vi "Tosca-Setup Schedule.vi"(0 "Tosca":refnum<class "Parameters.lvclass">) -> (4 "Tosca out":refnum<class "Parameters.lvclass">, 8 "Canceled?":bool)   [LabVIEW 2020]
uses:
  epl-vi-lib/Utility VIs/Controls/KTable/KTable.xctl
  epl-vi-lib/Utility VIs/Buttons/KCheckmarkBoolean 2.ctl
  epl-vi-lib/Utility VIs/Controls/KListboxEx/KListboxEx.xctl
  Classes/Parameters/Parameters.lvclass
  epl-vi-lib/Utility VIs/Controls/KTable/Events.ctl
  epl-vi-lib/Utility VIs/Controls/KTable/Event Data.ctl
  epl-vi-lib/Utility VIs/Controls/KTable/Event Type.ctl
  <vilib>/Utility/miscctls.llb/LVPoint32TypeDef.ctl
  epl-vi-lib/Utility VIs/Controls/KListboxEx/Event Action.ctl
  Typedefs/Tosca-Schedule Mode.ctl
  Classes/Parameters/Parameters.lvclass/Parameters.ctl
  Typedefs/Tosca-Adaptive Track.ctl
  Typedefs/Tosca-Simple Variable.ctl
  Adaptation VIs/Tosca-Adapt Threshold Metric.ctl
  Typedefs/Tosca-Parameter Family.ctl
  Typedefs/Tosca-Parameter Table Element.ctl
  Typedefs/Tosca-Parameter Dimension.ctl
  Typedefs/Tosca-Sequence Order.ctl
  Classes/Parameters/Read Schedule Mode.vi
  Classes/Parameters/Read Schedule.vi
  Classes/Parameters/Write Tracks.vi
  Classes/Parameters/Read Tracks.vi
  Classes/Parameters/Write Schedule Mode.vi
  Classes/Parameters/Write Schedule.vi
  Classes/Parameters/Read Families.vi
  Classes/Parameters/Write Families.vi
  Classes/Parameters/Read Adapt.vi
  Classes/Parameters/Write Adapt.vi
panel:
  in  "icon":u16(ring)
  in  "Mode":u16(ring) caption="Configure as" items=["Sequence", "CS+/CS-", "Adaptive track"]
  in  "OK":bool
  in  "Cancel":bool
  in  "Tab Control":enum32{"Schedule", "Adapt"}(tab)
  in  "browse":bool
  in  "Script":string
  in  "Update":bool
  in  "Balance":T1
  in  "order":u16(ring) items=["Sequential", "Alternate", "Randomized", "Random group", "Arbitrary"]
  in  "Family":u16(xcontrol)
  in  "Params":u16(xcontrol) caption="Parameters to vary for \"Item1\""
  out "Grid":i32[][](graph)
  in  "Blocks":i32 caption="Do this many blocks"
  in  "Test param":u16(xcontrol) caption="Test parameters"
  in  "switch type":enum16{"Trials", "Reversals"}(ring)
  in  "Switch after":i32
  in  "all catch":T1 caption="Do all catch"
  in  "Tracks":i32(xcontrol)
  in  "Pcatch":dbl caption="Probability of catch trial"
  in  "Adapt":T2={"mode"=enum."Add", "Step"="", "Start"=0.0, "Min"=0.0, "Max"=0.0, "Nup"=0, "Ndown"=0, "Nrev"=0, "compute"=enum."mean", "Ncompute"=0, "Step2"="", "change after"=1}
  in  "Catch parameters":u16(xcontrol) caption="Use 'A' for current value"
  in  "Adapt param":u16(xcontrol) caption="Stimulus"
  # "reversals"
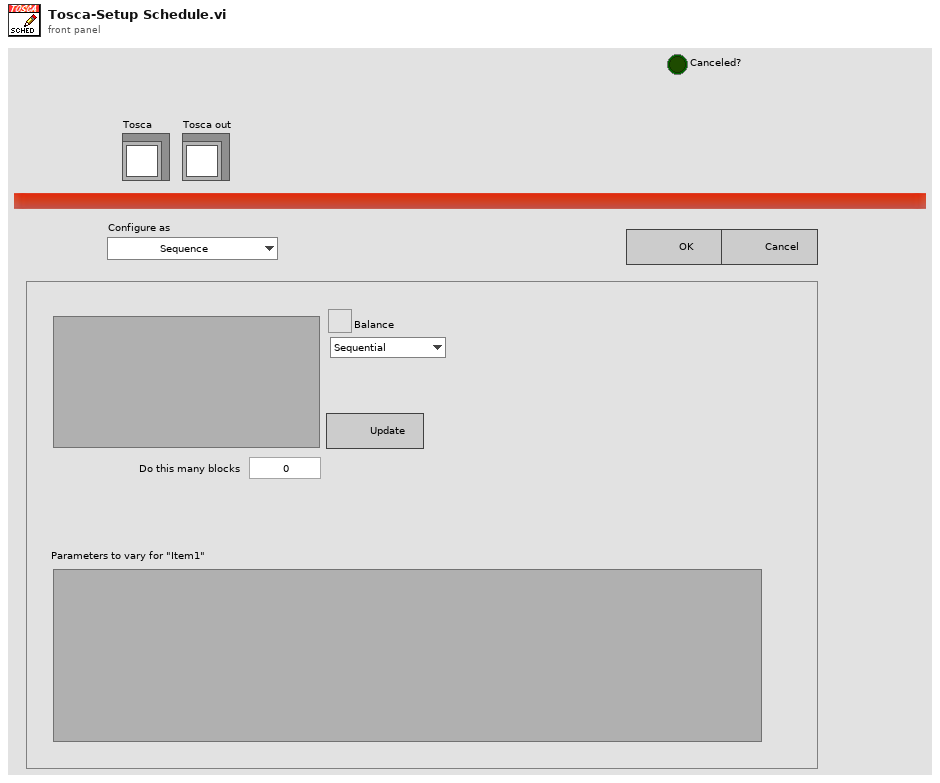
[diagram p1: front panel]
types:
  T1 = typedef "KCheckmarkBoolean 2.ctl" = bool
  T2 = cluster{"mode":enum16{"Add", "Multiply"}, "Step":string, "Start":dbl, "Min":dbl, "Max":dbl, "Nup":i32, "Ndown":i32, "Nrev":i32, "compute":enum16{"mean", "median"}, "Ncompute":i32, "Step2":string, "change after":i32}
  T3 = typedef "KTable.xctl/Events.ctl" = cluster{"Items Changed":refnum<user-event>}
  T4 = cluster{"Items Changed":refnum<user-event>, "List Changed":refnum<user-event>}
  T5 = typedef "LVPoint32TypeDef.ctl" = cluster{"Horizontal":i32, "Vertical":i32}
  T6 = cluster{"Coords":T5, "mouse":bool, "labels":string[][]}
  T7 = typedef "KListboxEx.xctl/Events.ctl" = cluster{"Items Changed":refnum<user-event>, "List Changed":refnum<user-event>}
  T8 = typedef "Tosca-Schedule Mode.ctl" = enum16{"Seq", "CS+/CS-", "Adapt"}
  T9 = typedef "Tosca-Adaptive Track.ctl" = cluster{"state":string, "chan":string, "param":string, "Start":dbl, "Step":string, "Mode":enum16{"Add", "Multiply"}, "Pcatch":dbl, "Ndown":i32, "Nup":i32, "Nreverse":i32, "Min":dbl, "Max":dbl, "Catch":T10[], "do all catch":bool, "name":string, "Vars":T10[], "compute":T11, "of last":i32, "Step2":string, "after":i32}
  T10 = typedef "Tosca-Simple Variable.ctl" = cluster{"state":string, "chan":string, "param":string, "expr":string}
  T11 = typedef "Tosca-Adapt Threshold Metric.ctl" = enum16{"mean", "median"}
  T12 = typedef "Tosca-Parameter Family.ctl" = cluster{"Name":string, "Number":i32, "Vars":T13[], "Mask":bool[][], "one each":bool}
  T13 = typedef "Tosca-Parameter Table Element.ctl" = cluster{"state":string, "chan":string, "param":string, "expr":string, "dim":T14, "value":dbl[]}
  T14 = typedef "Tosca-Parameter Dimension.ctl" = enum16{"Ind", "X", "Y"}
  T15 = typedef "Tosca-Sequence Order.ctl" = enum16{"Sequential", "Alternate", "Randomize", "Random group", "Arbitrary"}
  T16 = typedef "Tosca-Schedule.ctl" = cluster{"Blocks":i32, "order":T15, "balance":bool, "Families":T12[], "Script":path}
  T17 = typedef "KTable.xctl/Event Type.ctl" = enum16{"None", "Selection", "Edit", "Insert", "Delete", "Up", "Down", "Duplicate"}
  T18 = typedef "KListboxEx.xctl/Event Action.ctl" = enum16{"None", "Add", "Delete", "Move", "Edit", "Select"}
  T19 = typedef "Tosca-Adapt.ctl" = cluster{"Switch after":i32, "Switch type":enum16{"Trials", "Reversals"}, "Tracks":T9[]}
  T20 = cluster{"state":string, "chan":string, "param":string}[]
  T21 = cluster{"state":string, "chan":string, "param":string}
  T22 = cluster{"state":string, "chan":string, "param":string, "expr":string}[]
  T23 = cluster{"Name":string, "Number":i32, "one each":bool}
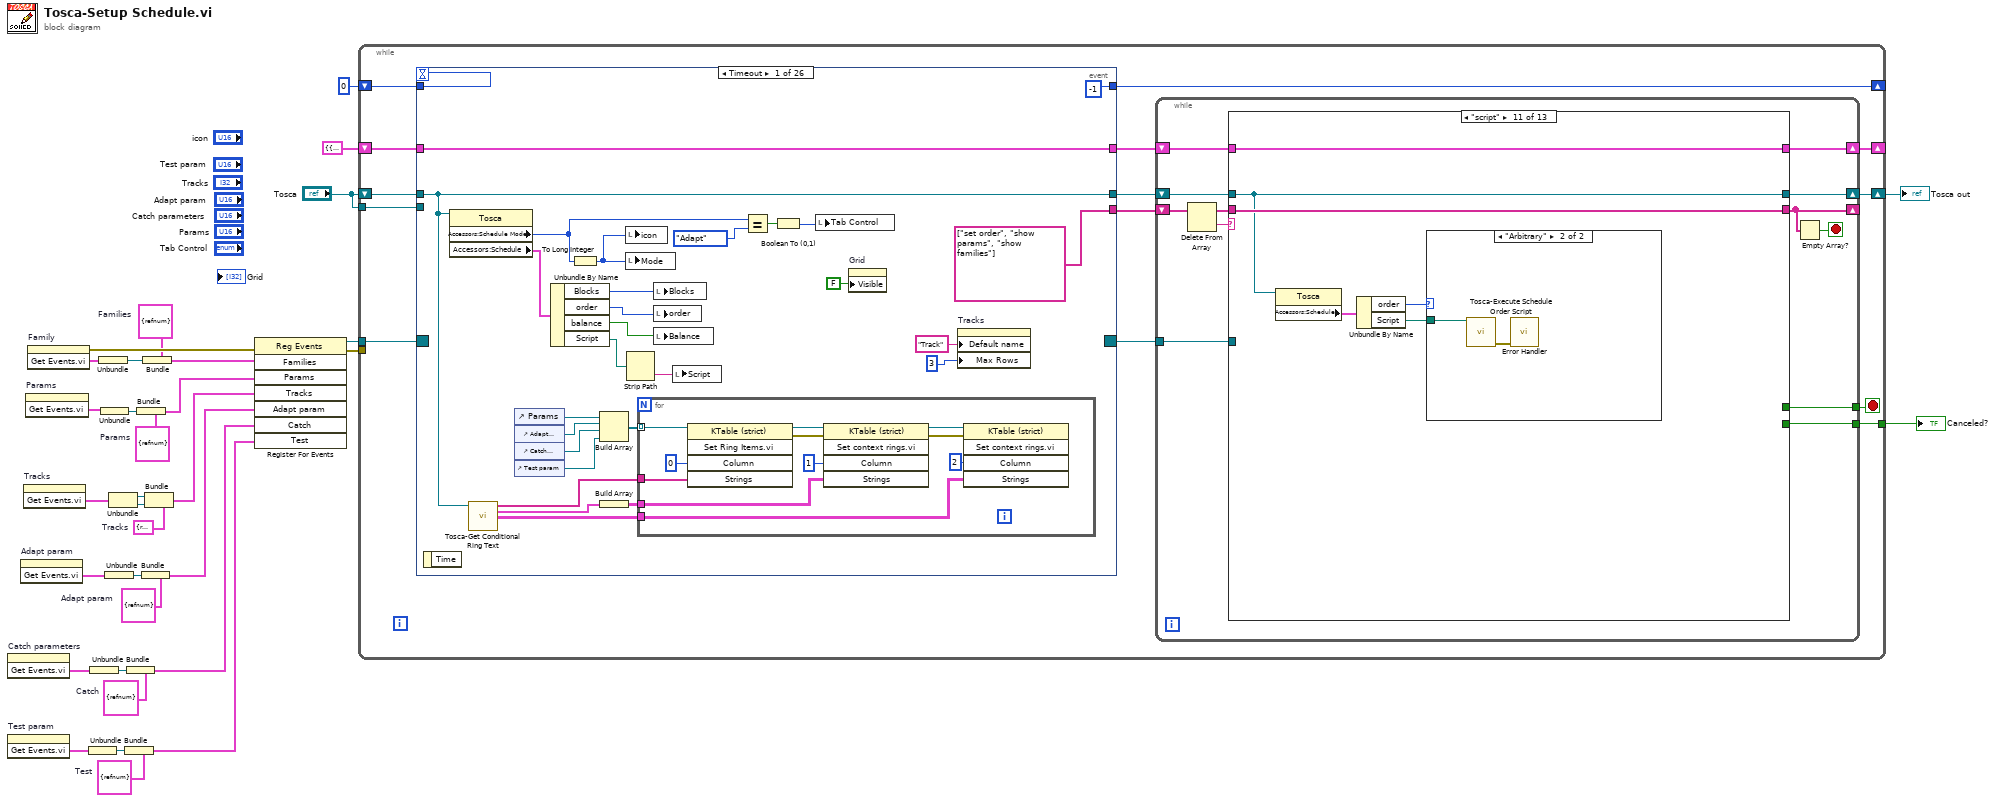
[diagram p0: block diagram]
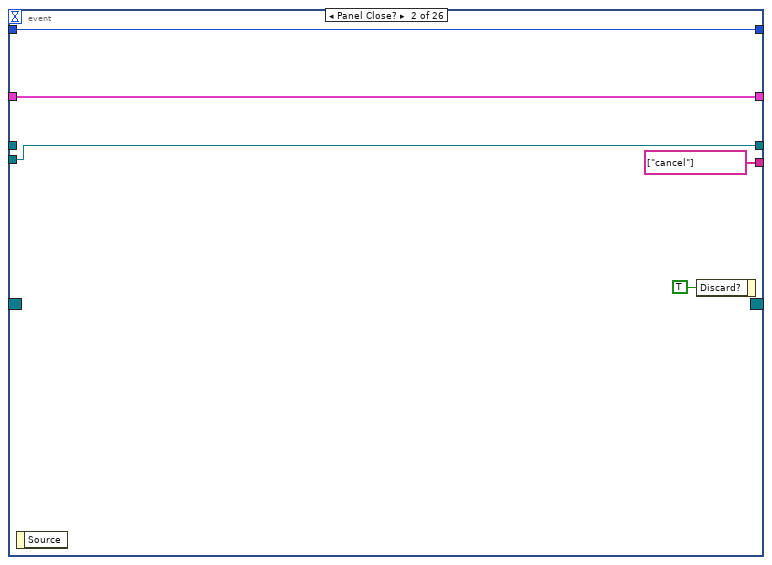
[diagram p2: hidden frame]
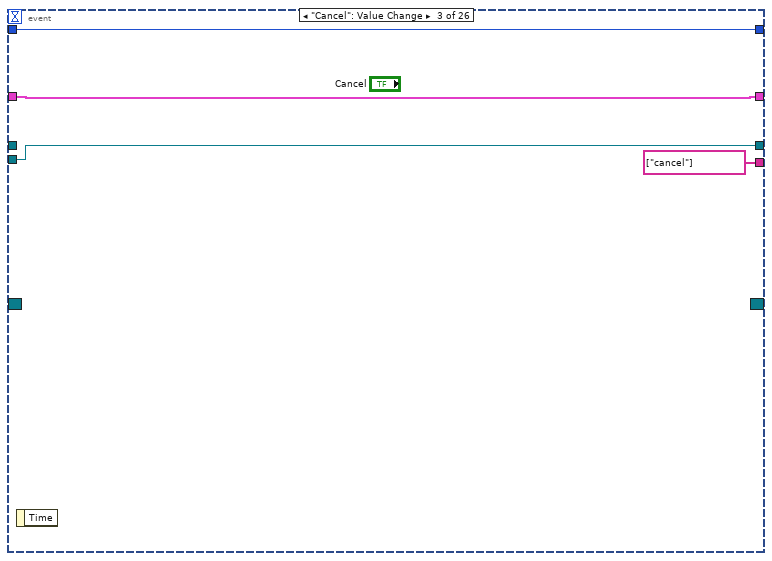
[diagram p3: hidden frame]
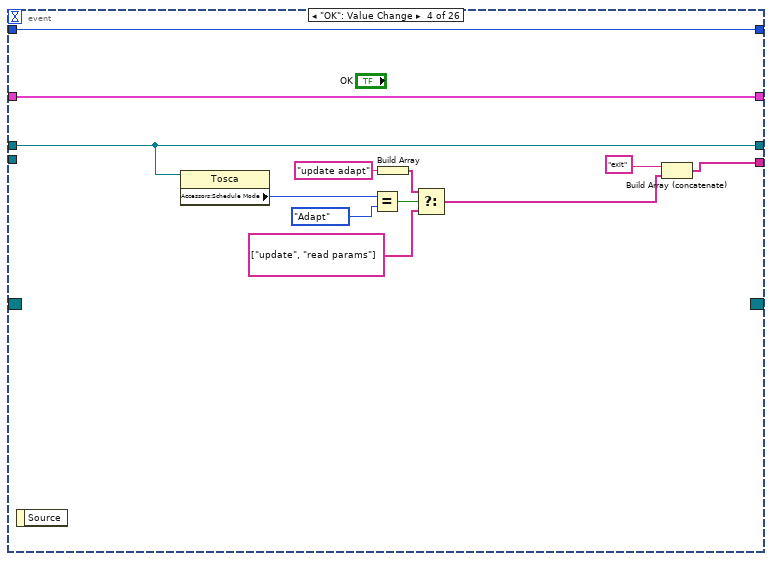
[diagram p4: hidden frame]
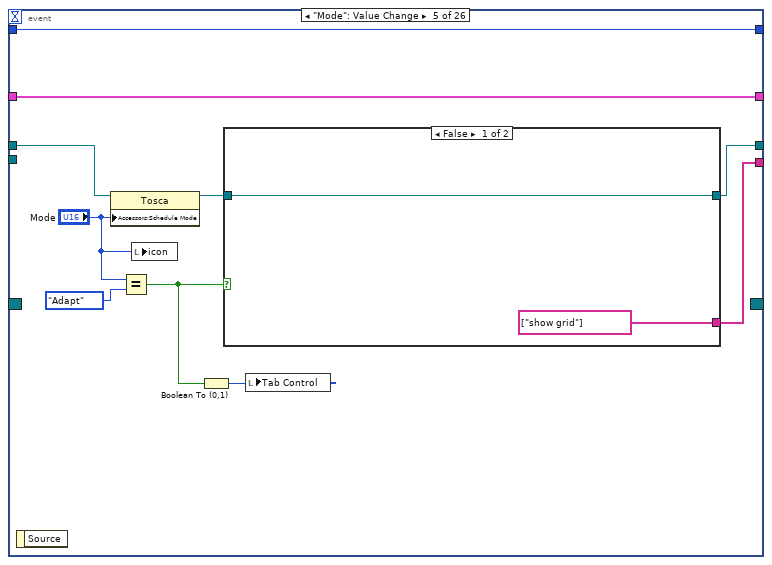
[diagram p5: hidden frame]
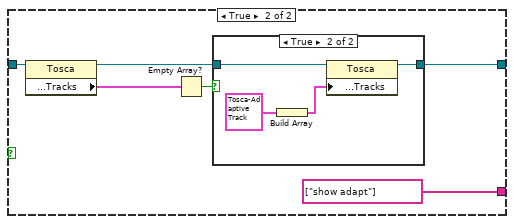
[diagram p6: hidden frame]
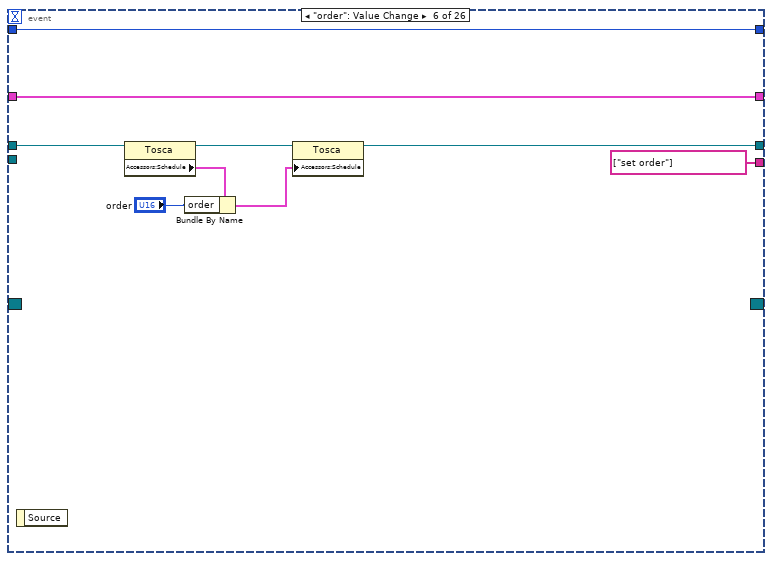
[diagram p8: hidden frame]
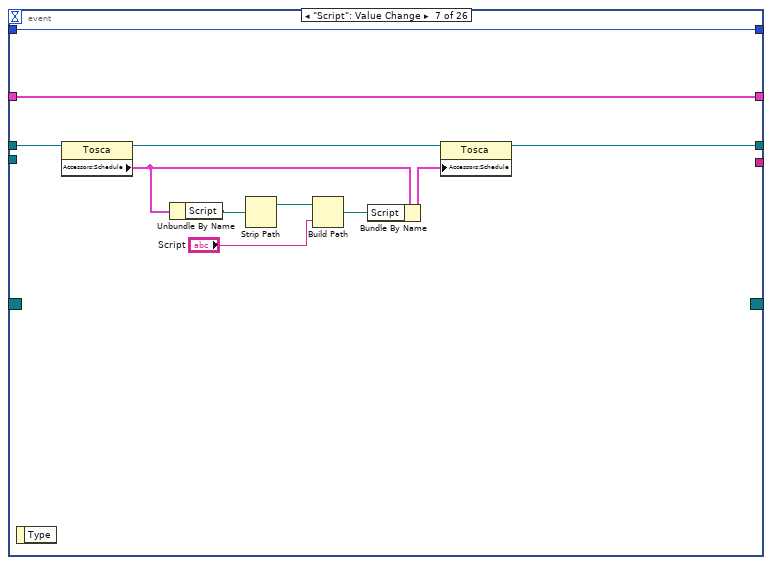
[diagram p9: hidden frame]
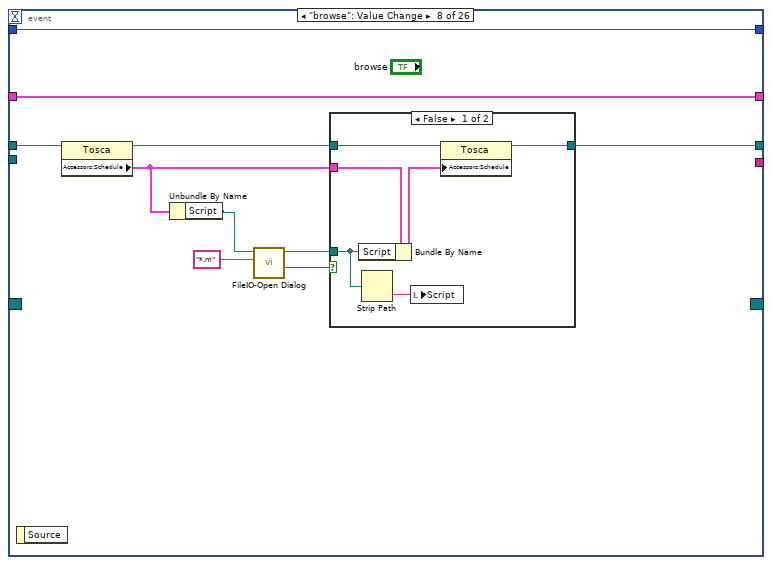
[diagram p10: hidden frame]
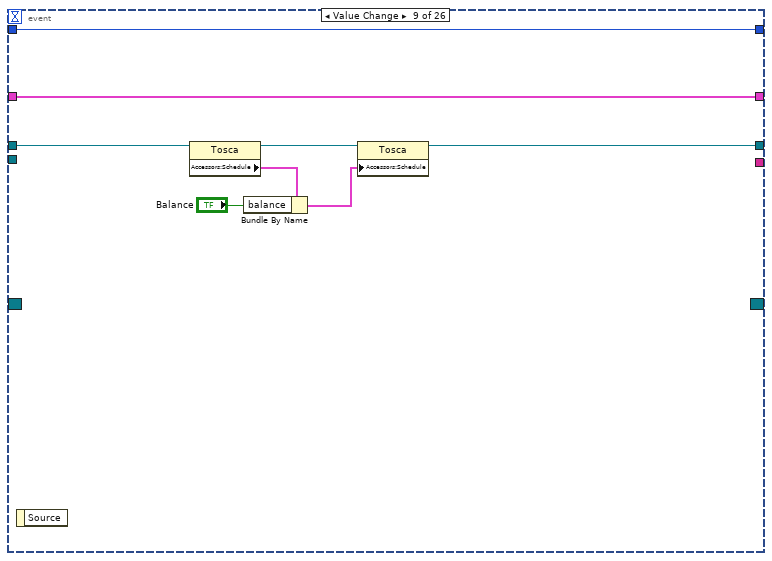
[diagram p12: hidden frame]
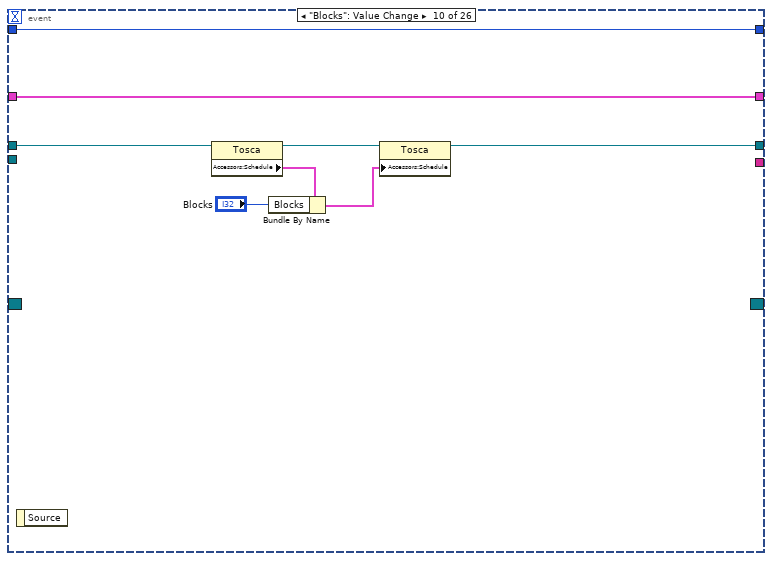
[diagram p13: hidden frame]
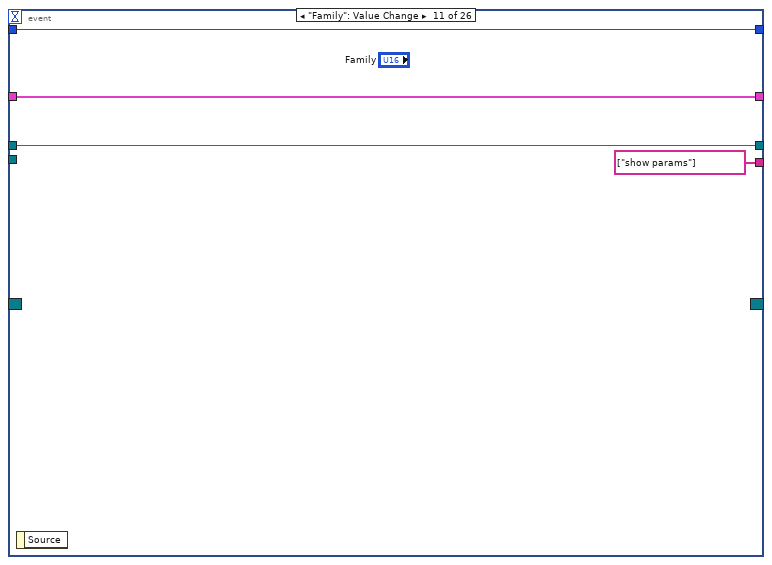
[diagram p14: hidden frame]
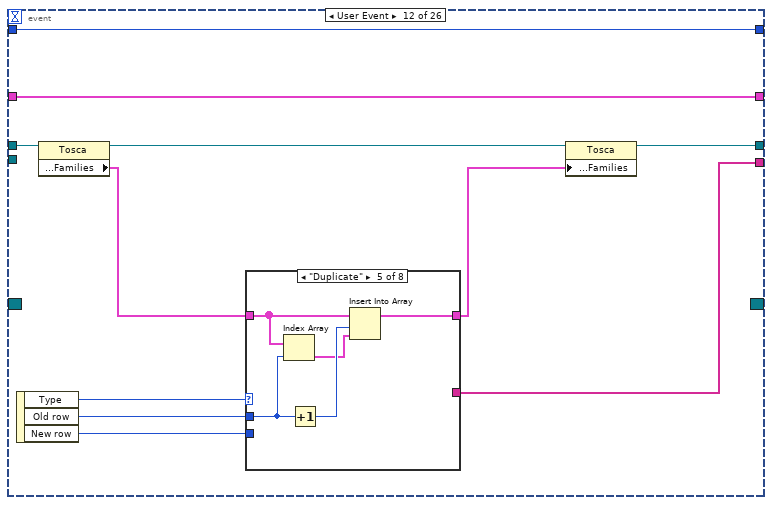
[diagram p15: hidden frame]
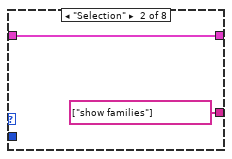
[diagram p17: hidden frame]
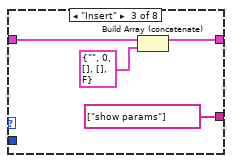
[diagram p18: hidden frame]
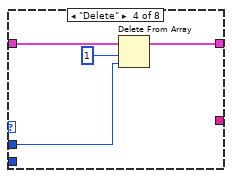
[diagram p19: hidden frame]
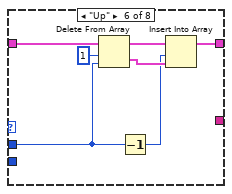
[diagram p20: hidden frame]
diagram:
  w7 = T3 {"Items Changed"=refnum}  # Test
  w10 = T3 {"Items Changed"=refnum}  # Catch
  w14 = T3 {"Items Changed"=refnum}  # Adapt param
  w17 = T4 {"Items Changed"=refnum, "List Changed"=refnum}  # Tracks
  w24 = T3 {"Items Changed"=refnum}  # Params
  w30 = T3 {"Items Changed"=refnum}  # Families
  n1 = invoke on="Catch parameters" class="KTable (strict)" method="Get Events.vi"() -> ("Get Events.vi"=w11:T3)  [unwired: 3 in, 2 out]
  n2 = invoke on="Test param" class="KTable (strict)" method="Get Events.vi"() -> ("Get Events.vi"=w6:T3)  [unwired: 3 in, 2 out]
  n3 = invoke on="Adapt param" class="KTable (strict)" method="Get Events.vi"() -> ("Get Events.vi"=w15:T3)  [unwired: 3 in, 2 out]
  n4 = invoke on="Tracks" class="KListboxEx (strict)" method="Get Events.vi"() -> ("Get Events.vi"=w20:T7)  [unwired: 3 in, 2 out]
  n5 = invoke on="Params" class="KTable (strict)" method="Get Events.vi"() -> ("Get Events.vi"=w25:T3)  [unwired: 3 in, 2 out]
  n6 = invoke on="Family" class="KTable (strict)" method="Get Events.vi"() -> (error out=w31:errorcluster, "Get Events.vi"=w29:T3)  [unwired: 3 in, 1 out]
  n7 = Unbundle(w6) -> ("Items Changed"=w8:refnum<user-event>)
  n8 = Unbundle(w11) -> ("Items Changed"=w12:refnum<user-event>)
  n9 = Unbundle(w29) -> ("Items Changed"=w28:refnum<user-event>)
  n10 = Unbundle(w25) -> ("Items Changed"=w26:refnum<user-event>)
  n11 = Unbundle(w15) -> ("Items Changed"=w16:refnum<user-event>)
  n12 = Unbundle(w20) -> ("Items Changed"=w21:refnum<user-event>, "List Changed"=w19:refnum<user-event>)
  n13 = Bundle(cluster=w7, "Items Changed"=w8) -> (w5:T3)
  n14 = Bundle(cluster=w10, "Items Changed"=w12) -> (w9:T3)
  n15 = Bundle(cluster=w24, "Items Changed"=w26) -> (w23:T3)
  n16 = Bundle(cluster=w14, "Items Changed"=w16) -> (w13:T3)
  n17 = Bundle(cluster=w30, "Items Changed"=w28) -> (w27:T3)
  n18 = Bundle(cluster=w17, "Items Changed"=w21, "List Changed"=w19) -> (w18:T4)
  n19 = register-events(error in=w31, w27, w23, w18, w13, w9, w5) -> (reference out=w1:refnum<event-registration>, error out=w2:errorcluster)  [unwired: 1 in]
  n20 = while {
    shift-right: [w47] -> _
    shift-left: 0 -> [w46]
    tunnel: [w39] -> w32
    shift-right: [w41] -> w3
    shift-left: "Tosca" -> [w45]
    tunnel: "Tosca" -> [w44]
    shift-right: [w36] -> _
    shift-left: T6 {"Coords"={"Horizontal"=0, "Vertical"=0}, "mouse"=FALSE, "labels"=[]} -> [w38]
    tunnel: w2 -> [_]
    tunnel: w1 -> [w35]
    stop <- w40 stop-if-true
    n21 = event shown="[0] Timeout" {
      selector: w35 -> [_ _ _ _ _ _ _ _ _ _ _ _ _ _ _ _ _ _ _ _ _ _ _ _ _ _]
      dyn-events: [_ _ _ _ _ _ _ _ _ _ _ _ _ _ _ _ _ _ _ _ _ _ _ _ _ _] -> w34
      timeout: w46 -> [_ _ _ _ _ _ _ _ _ _ _ _ _ _ _ _ _ _ _ _ _ _ _ _ _ _]
      tunnel: [-1 w90 w94 w106 w116 w138 w149 w159 w174 w182 w186 w197 w241 w284 w299 w314 w336 w373 w382 w390 w414 w425 w442 w455 w468 w479] -> w47
      tunnel: w46 -> [_ w90 w94 w106 w116 w138 w149 w159 w174 w182 w186 w197 w241 w284 w299 w314 w336 w373 w382 w390 w414 w425 w442 w455 w468 w479]
      tunnel: w45 -> [w50 _ _ w96 w110 w135 w147 w157 w169 w176 w185 w190 w234 w283 w296 w304 w329 w367 w379 w384 w395 w419 w430 w447 w460 w473]
      tunnel: [w50 w86 w93 w96 w107 w131 w140 w154 w168 w175 w185 w189 w233 w283 w296 w303 w325 w366 w377 w383 w394 w418 w428 w446 w459 w472] -> w43
      tunnel: w44 -> [_ w86 w93 _ _ _ _ _ _ _ _ _ _ _ _ _ _ _ _ _ _ _ _ _ _ _]
      tunnel: [string[] ["set order", "show params", "show families"] string[] ["cancel"] string[] ["cancel"] w102 w112 string[] ["set order"] _ _ _ _ string[] ["show params"] w193 w237 string[] ["script", "update", "read params"] _ _ w330 w371 _ _ _ _ _ _ _ _] -> w42
      tunnel: w38 -> [w66 w89 w91 w105 w115 w136 w148 w158 w173 w181 w184 w192 w235 w281 w291 w305 w335 w372 w381 w389 w413 w424 w441 w454 w467 w478]
      tunnel: [w66 w89 w91 w105 w115 w136 w148 w158 w173 w181 w184 w192 w235 w281 w289 w305 w335 w372 w381 w389 w413 w424 w441 w454 w467 w478] -> w37
      event Timeout {
        n22 = event-data() -> ()  [unwired: 1 in, 1 out]
        n23 = property class="Tosca"(reference=w50) -> ("Accessors:Schedule Mode"=w51:T8, "Accessors:Schedule"=w52:T16)  [unwired: 1 in, 2 out]
        n24 = call "Tosca-Get Conditional Ring Text.vi"("Tosca"=w50) -> ("States"=w53:string[], "StimChans"=w73:cluster{string[]}[], "Params"=w71:cluster{"Parameter Names":string[]}[][])  [unwired: 12 in]
        n25 = control-ref of="Params"() -> (w60:refnum<vi>)
        n26 = control-ref of="Adapt param"() -> (w59:refnum<vi>)
        n27 = control-ref of="Catch parameters"() -> (w58:refnum<vi>)
        n28 = control-ref of="Test param"() -> (w54:refnum<vi>)
        n29 = Unbundle By Name(w52) -> ("Blocks"=w70:i32, "order"=w69:T15, "balance"=w68:bool, "Script"=w49:path)
        n30 = To Long Integer(number=w51) -> (32bit integer=w65:i32)
        n31 = Build Array(w60, w59, w58, w54) -> (w57:refnum<vi>[])
        n32 = Build Array(w73) -> (w72:cluster{string[]}[][])
        n33 = local write "icon"(w65) -> ()
        n34 = local write "Mode"(w65) -> ()
        n35 = Strip Path(path=w49) -> (name=w48:string)  [unwired: 1 out]
        n36 = for {
          tunnel: w72 -> [w80]
          tunnel: w71 -> [w79]
          tunnel: w53 -> [w78]
          tunnel: w57 -> [w75] mode=indexing
          n37 = invoke on="Invoke Node" class="KTable (strict)" method="Set Ring Items.vi"(reference=w75, "Column"=0, "Strings"=w78) -> (reference out=w77:refnum<vi>, error out=w83:errorcluster)  [unwired: 2 in, 3 out]
          n38 = invoke on="Invoke Node" class="KTable (strict)" method="Set context rings.vi"(reference=w77, error in=w83, "Column"=1, "Strings"=w80) -> (reference out=w76:refnum<vi>, error out=w82:errorcluster)  [unwired: 1 in, 3 out]
          n39 = invoke on="Invoke Node" class="KTable (strict)" method="Set context rings.vi"(reference=w76, error in=w82, "Column"=2, "Strings"=w79) -> ()  [unwired: 1 in, 5 out]
        }
        n40 = local write "Blocks"(w70) -> ()
        n41 = local write "order"(w69) -> ()
        n42 = local write "Balance"(w68) -> ()
        n43 = local write "Script"(w48) -> ()
        n44 = Equal?(x=w51, y=Tosca-Schedule_Mode."Adapt") -> (x = y?=w63:bool)
        n45 = Boolean To (0,1)(Boolean=w63) -> (0, 1=w62:i16)
        n46 = local write "Tab Control"(w62) -> ()
        n47 = property on="Grid" class="IntGraph (strict)"("Visible"=FALSE) -> ()  [unwired: 2 in, 2 out]
        n48 = property on="Tracks" class="KListboxEx (strict)"("Default name"="Track", "Max Rows"=3) -> ()  [unwired: 2 in, 2 out]
      }
      event Panel Close? {
        n49 = event-data() -> ()  [unwired: 1 in, 1 out]
        n50 = event-data("Discard?"=TRUE) -> ()  [unwired: 1 in, 1 out]
      }
      event "Cancel": Value Change {
        n51 = event-data() -> ()  [unwired: 1 in, 1 out]
      }
      event "OK": Value Change {
        n52 = event-data() -> ()  [unwired: 1 in, 1 out]
        n53 = property class="Tosca"(reference=w96) -> ("Accessors:Schedule Mode"=w95:T8)  [unwired: 1 in, 2 out]
        n54 = Equal?(x=w95, y=Tosca-Schedule_Mode."Adapt") -> (x = y?=w100:bool)
        n55 = Build Array("update adapt" ("t")) -> (w98:string[])
        n56 = Select(t=w98, s=w100, f=string[] ["update", "read params"]) -> (s? t:f=w103:string[])
        n57 = Build Array (concatenate)("exit", w103) -> (w102:string[])
      }
      event "Mode": Value Change {
        n58 = event-data() -> ()  [unwired: 1 in, 1 out]
        n59 = property class="Tosca"(reference=w110, "Accessors:Schedule Mode"="Mode") -> (reference out=w108:refnum<class "Parameters.lvclass">)  [unwired: 1 in, 1 out]
        n60 = Equal?(x="Mode", y=Tosca-Schedule_Mode."Adapt") -> (x = y?=w113:bool)
        n61 = local write "icon"("Mode") -> ()
        n62 = Boolean To (0,1)(Boolean=w113) -> (0, 1=w114:i16)
        n63 = case shown="False" w113 {
          tunnel: [string[] ["show grid"] string[] ["show adapt"]] -> w112
          tunnel: w108 -> [w117 w122]
          tunnel: [w117 w119] -> w107
          frame False {
          }
          frame True {
            n64 = property class="Tosca"(reference=w122) -> (reference out=w120:refnum<class "Parameters.lvclass">, "Accessors:Adapt.Tracks"=w121:T9[])  [unwired: 1 in, 1 out]
            n65 = Empty Array?(array=w121) -> (empty?=w123:bool)
            n66 = case shown="True" w123 {
              tunnel: w120 -> [w125 w128]
              tunnel: [w125 w127] -> w119
              frame False {
              }
              frame True {
                n67 = Build Array(T9 {"state"="", "chan"="", "param"="", "Start"=90.0, "Step"="-5", "Mode"=enum."Add", "Pcatch"=100.0, "Ndown"=2, "Nup"=1, "Nreverse"=6, "Min"=0.0, "Max"=100.0, "Catch"=[], "do all catch"=FALSE, "name"="Track1", "Vars"=[], "compute"=enum."mean", "of last"=0, "Step2"="", "after"=0} ("Track")) -> (w126:T9[])
                n68 = property class="Tosca"(reference=w128, "Accessors:Adapt.Tracks"=w126) -> (reference out=w127:refnum<class "Parameters.lvclass">)  [unwired: 1 in, 1 out]
              }
            }
          }
        }
        n69 = local write "Tab Control"(w114) -> ()
      }
      event "order": Value Change {
        n70 = event-data() -> ()  [unwired: 1 in, 1 out]
        n71 = property class="Tosca"(reference=w135) -> (reference out=w133:refnum<class "Parameters.lvclass">, "Accessors:Schedule"=w134:T16)  [unwired: 1 in, 1 out]
        n72 = Bundle By Name(cluster=w134, "order"="order") -> (w132:T16)
        n73 = property class="Tosca"(reference=w133, "Accessors:Schedule"=w132) -> (reference out=w131:refnum<class "Parameters.lvclass">)  [unwired: 1 in, 1 out]
      }
      event "Script": Value Change {
        n74 = event-data() -> ()  [unwired: 1 in, 1 out]
        n75 = property class="Tosca"(reference=w147) -> (reference out=w141:refnum<class "Parameters.lvclass">, "Accessors:Schedule"=w143:T16)  [unwired: 1 in, 1 out]
        n76 = Unbundle By Name(w143) -> ("Script"=w146:path)
        n77 = Strip Path(path=w146) -> (stripped path=w145:path)  [unwired: 1 out]
        n78 = Build Path(base path=w145, name or relative path="Script") -> (appended path=w142:path)
        n79 = Bundle By Name(cluster=w143, "Script"=w142) -> (w139:T16)
        n80 = property class="Tosca"(reference=w141, "Accessors:Schedule"=w139) -> (reference out=w140:refnum<class "Parameters.lvclass">)  [unwired: 1 in, 1 out]
      }
      event "browse": Value Change {
        n81 = event-data() -> ()  [unwired: 1 in, 1 out]
        n82 = property class="Tosca"(reference=w157) -> (reference out=w155:refnum<class "Parameters.lvclass">, "Accessors:Schedule"=w156:T16)  [unwired: 1 in, 1 out]
        n83 = Unbundle By Name(w156) -> ("Script"=w153:path)
        n84 = call "FileIO-Open Dialog.vi"("pattern (all files)"="*.m", "Start path"=w153) -> ("cancelled"=w151:bool, "selected path"=w150:path)  [unwired: 7 in, 1 out]
        n85 = case shown="False" w151 {
          tunnel: w156 -> [w165 _]
          tunnel: w155 -> [w164 w166]
          tunnel: [w163 w166] -> w154
          tunnel: w150 -> [w161 _]
          frame False {
            n86 = Bundle By Name(cluster=w165, "Script"=w161) -> (w162:T16)
            n87 = Strip Path(path=w161) -> (name=w160:string)  [unwired: 1 out]
            n88 = local write "Script"(w160) -> ()
            n89 = property class="Tosca"(reference=w164, "Accessors:Schedule"=w162) -> (reference out=w163:refnum<class "Parameters.lvclass">)  [unwired: 1 in, 1 out]
          }
          frame True {
          }
        }
      }
      event Value Change {
        n90 = event-data() -> ()  [unwired: 1 in, 1 out]
        n91 = property class="Tosca"(reference=w169) -> (reference out=w171:refnum<class "Parameters.lvclass">, "Accessors:Schedule"=w172:T16)  [unwired: 1 in, 1 out]
        n92 = Bundle By Name(cluster=w172, "balance"="Balance") -> (w170:T16)
        n93 = property class="Tosca"(reference=w171, "Accessors:Schedule"=w170) -> (reference out=w168:refnum<class "Parameters.lvclass">)  [unwired: 1 in, 1 out]
      }
      event "Blocks": Value Change {
        n94 = event-data() -> ()  [unwired: 1 in, 1 out]
        n95 = property class="Tosca"(reference=w176) -> (reference out=w179:refnum<class "Parameters.lvclass">, "Accessors:Schedule"=w180:T16)  [unwired: 1 in, 1 out]
        n96 = Bundle By Name(cluster=w180, "Blocks"="Blocks") -> (w178:T16)
        n97 = property class="Tosca"(reference=w179, "Accessors:Schedule"=w178) -> (reference out=w175:refnum<class "Parameters.lvclass">)  [unwired: 1 in, 1 out]
      }
      event "Family": Value Change {
        n98 = event-data() -> ()  [unwired: 1 in, 1 out]
      }
      event User Event {
        n99 = event-data() -> ("Type"=w196:T17, "Old row"=w195:i32, "New row"=w194:i32)  [unwired: 1 in]
        n100 = property class="Tosca"(reference=w190) -> (reference out=w191:refnum<class "Parameters.lvclass">, "Accessors:Schedule.Families"=w188:T12[])  [unwired: 1 in, 1 out]
        n101 = case shown="\"Duplicate\"" w196 {
          tunnel: w195 -> [_ _ _ w207 w213 w218 w225 _]
          tunnel: [w198 w200 w204 w205 w211 w214 w221 w229] -> w187
          tunnel: w194 -> [_ _ _ _ _ _ _ _]
          tunnel: w188 -> [w198 w200 w203 w206 w212 w216 w223 w229]
          tunnel: [_ string[] ["show families"] string[] ["show params"] _ _ _ _ string[] ["show params", "read families"]] -> w193
          frame "None", Default {
          }
          frame "Selection" {
          }
          frame "Insert" {
            n102 = Build Array (concatenate)(w203, T12 {"Name"="", "Number"=0, "Vars"=[], "Mask"=[], "one each"=FALSE} ("Family")) -> (w204:T12[])
          }
          frame "Delete" {
            n103 = Delete From Array(array=w206, length=1, index=w207) -> (array with subset deleted=w205:T12[])  [unwired: 1 out]
          }
          frame "Duplicate" {
            n104 = Index Array(array=w212, index=w213) -> (element=w209:T12)
            n105 = Increment(x=w213) -> (x+1=w210:i32)
            n106 = Insert Into Array(array=w212, index=w210, new element=w209) -> (w211:T12[])
          }
          frame "Up" {
            n107 = Delete From Array(array=w216, length=1, index=w218) -> (deleted portion=w219:T12[], array with subset deleted=w215:T12[])
            n108 = Decrement(x=w218) -> (x-1=w217:i32)
            n109 = Insert Into Array(array=w215, index=w217, new element=w219) -> (w214:T12[])
          }
          frame "Down" {
            n110 = Delete From Array(array=w223, length=1, index=w225) -> (deleted portion=w226:T12[], array with subset deleted=w222:T12[])
            n111 = Increment(x=w225) -> (x+1=w224:i32)
            n112 = Insert Into Array(array=w222, index=w224, new element=w226) -> (w221:T12[])
          }
          frame "Edit" {
          }
        }
        n113 = property class="Tosca"(reference=w191, "Accessors:Schedule.Families"=w187) -> (reference out=w189:refnum<class "Parameters.lvclass">)  [unwired: 1 in, 1 out]
      }
      event User Event {
        n114 = event-data() -> ("Type"=w240:T17, "Old row"=w239:i32, "New row"=w238:i32)  [unwired: 1 in]
        n115 = property class="Tosca"(reference=w234) -> (reference out=w232:refnum<class "Parameters.lvclass">, "Accessors:Schedule.Families"=w231:T12[])  [unwired: 1 in, 1 out]
        n116 = local read "Family"() -> (w236:u16)
        n117 = in-place {
          in-place-border: w240 -> [w249]
          in-place-border: w239 -> [w248]
          in-place-border: w238 -> [w247]
          in-place-border: [w246] -> w237
          n118 = in-place-array #1(w231, w236) -> (w243:T12)
          n119 = Unbundle By Name(w243) -> ("Vars"=w245:T13[])
          n120 = case shown="\"Duplicate\"" w249 {
            tunnel: w248 -> [_ _ _ w257 w262 w269 w276 _]
            tunnel: [w250 w251 w254 w255 w260 w265 w272 w280] -> w244
            tunnel: w247 -> [_ _ _ _ _ _ _ _]
            tunnel: w245 -> [w250 w251 w253 w256 w261 w267 w274 w280]
            tunnel: [_ _ _ _ string[] ["show params"] _ _ string[] ["read params"]] -> w246
            frame "None", Default {
            }
            frame "Selection" {
            }
            frame "Insert" {
              n121 = Build Array (concatenate)(w253, T13 {"state"="", "chan"="", "param"="", "expr"="", "dim"=enum."Ind", "value"=[]} ("Array")) -> (w254:T13[])
            }
            frame "Delete" {
              n122 = Delete From Array(array=w256, length=1, index=w257) -> (array with subset deleted=w255:T13[])  [unwired: 1 out]
            }
            frame "Duplicate" {
              n123 = Index Array(array=w261, index=w262) -> (element=w263:T13)
              n124 = Increment(x=w262) -> (x+1=w264:i32)
              n125 = Insert Into Array(array=w261, index=w264, new element=w263) -> (w260:T13[])
            }
            frame "Up" {
              n126 = Delete From Array(array=w267, length=1, index=w269) -> (deleted portion=w270:T13[], array with subset deleted=w266:T13[])
              n127 = Decrement(x=w269) -> (x-1=w268:i32)
              n128 = Insert Into Array(array=w266, index=w268, new element=w270) -> (w265:T13[])
            }
            frame "Down" {
              n129 = Delete From Array(array=w274, length=1, index=w276) -> (deleted portion=w277:T13[], array with subset deleted=w273:T13[])
              n130 = Increment(x=w276) -> (x+1=w275:i32)
              n131 = Insert Into Array(array=w273, index=w275, new element=w277) -> (w272:T13[])
            }
            frame "Edit" {
            }
          }
          n132 = Bundle By Name(cluster=w243, "Vars"=w244) -> (w242:T12)
          n133 = in-place-array #1(w242) -> (w230:T12[])  [unwired: 1 out]
        }
        n134 = property class="Tosca"(reference=w232, "Accessors:Schedule.Families"=w230) -> (reference out=w233:refnum<class "Parameters.lvclass">)  [unwired: 1 in, 1 out]
      }
      event "Update": Value Change {
        n135 = event-data() -> ()  [unwired: 1 in, 1 out]
      }
      event "Grid": Mouse Move {
        n136 = event-data() -> ("CtlRef"=w298:refnum<vi>, "Coords"=w297:T5)  [unwired: 1 in]
        n137 = Unbundle By Name(w291) -> ("labels"=w290:string[][])
        n138 = invoke class="IntGraph (strict)" method="Map Coords To XY"(reference=w298, "Coords"=w297) -> ("XY"=w293:cluster{"X":dbl, "Y":dbl})  [unwired: 5 in, 6 out]
        n139 = Round Toward -Infinity(1:w293) -> (0:w294:cluster{"X":dbl, "Y":dbl})
        n140 = Max & Min(x=w294, y=0) -> (max(x,y)=w295:cluster{"X":dbl, "Y":dbl})  [unwired: 1 out]
        n141 = To Long Integer(number=w295) -> (32bit integer=w288:cluster{"X":i32, "Y":i32})
        n142 = Unbundle(w288) -> ("X"=w287:i32, "Y"=w286:i32)
        n143 = Index Array(array=w290, index (row)=w287, index (col)=w286) -> (element=w285:string)
        n144 = Bundle By Name(cluster=w291, "Coords"=w288) -> (w289:T6)
        n145 = property on="Grid" class="IntGraph (strict)"("Caption.Text"=w285) -> ()  [unwired: 2 in, 2 out]
      }
      event "Grid": Mouse Down {
        n146 = event-data() -> ("CtlRef"=w310:refnum<vi>, "Coords"=w309:T5)  [unwired: 1 in]
        n147 = property class="Tosca"(reference=w304) -> (reference out=w302:refnum<class "Parameters.lvclass">, "Accessors:Schedule.Families"=w301:T12[])  [unwired: 1 in, 1 out]
        n148 = local read "Family"() -> (w306:u16)
        n149 = invoke class="IntGraph (strict)" method="Map Coords To XY"(reference=w310, "Coords"=w309) -> ("XY"=w308:cluster{"X":dbl, "Y":dbl})  [unwired: 5 in, 6 out]
        n150 = Round Toward -Infinity(1:w308) -> (0:w311:cluster{"X":dbl, "Y":dbl})
        n151 = Max & Min(x=w311, y=0) -> (max(x,y)=w313:cluster{"X":dbl, "Y":dbl})  [unwired: 1 out]
        n152 = To Long Integer(number=w313) -> (32bit integer=w307:cluster{"X":i32, "Y":i32})
        n153 = in-place {
          in-place-border: w307 -> [w324]
          n154 = in-place-array #2(w301, w306) -> (w316:T12)
          n155 = Unbundle By Name(w316) -> ("Mask"=w322:bool[][])
          n156 = Unbundle(w324) -> ("X"=w319:i32, "Y"=w320:i32)
          n157 = Index Array(array=w322, index (row)=w319, index (col)=w320) -> (element=w323:bool)
          n158 = Not(x=w323) -> (.not. x?=w321:bool)
          n159 = Replace Array Subset(array=w322, new element=w321, index (row)=w319, index (col)=w320) -> (w318:bool[][])
          n160 = Bundle By Name(cluster=w316, "Mask"=w318) -> (w315:T12)
          n161 = Boolean To (0,1)(Boolean=w318) -> (0, 1=w317:i16[][])
          n162 = local write "Grid"(w317) -> ()
          n163 = in-place-array #2(w315) -> (w300:T12[])  [unwired: 1 out]
        }
        n164 = property class="Tosca"(reference=w302, "Accessors:Schedule.Families"=w300) -> (reference out=w303:refnum<class "Parameters.lvclass">)  [unwired: 1 in, 1 out]
      }
      event User Event {
        n165 = event-data() -> ("Action"=w334:T18, "Name"=w332:string, "Start row"=w333:i32, "End row"=w331:i32)  [unwired: 1 in]
        n166 = property class="Tosca"(reference=w329) -> (reference out=w326:refnum<class "Parameters.lvclass">, "Accessors:Adapt.Tracks"=w328:T9[])  [unwired: 1 in, 1 out]
        n167 = case shown="\"Move\"" w334 {
          tunnel: w328 -> [w337 w339 w349 w353 w360]
          tunnel: [w337 w338 w348 w352 w359] -> w327
          tunnel: w333 -> [_ w343 w350 w357 w362]
          tunnel: w332 -> [_ w345 _ _ w363]
          tunnel: w331 -> [_ _ _ w354 _]
          tunnel: [_ string[] ["show track"] _ _ _] -> w330
          frame "None", Default {
          }
          frame "Add" {
            n168 = Decrement(x=w343) -> (x-1=w347:i32)
            n169 = Max & Min(x=0, y=w347) -> (max(x,y)=w340:i32)  [unwired: 1 out]
            n170 = Index Array(array=w339, index=w340) -> (element=w346:T9)
            n171 = Bundle By Name(cluster=w346, "name"=w345) -> (w342:T9)
            n172 = Insert Into Array(array=w339, index=w343, new element=w342) -> (w338:T9[])
            n173 = local write "Tracks"(w343) -> ()
          }
          frame "Delete" {
            n174 = Delete From Array(array=w349, length=1, index=w350) -> (array with subset deleted=w348:T9[])  [unwired: 1 out]
          }
          frame "Move" {
            n175 = Delete From Array(array=w353, length=1, index=w357) -> (deleted portion=w355:T9[], array with subset deleted=w356:T9[])
            n176 = Insert Into Array(array=w356, index=w354, new element=w355) -> (w352:T9[])
          }
          frame "Edit" {
            n177 = Index Array(array=w360, index=w362) -> (element=w364:T9)
            n178 = Bundle By Name(cluster=w364, "name"=w363) -> (w361:T9)
            n179 = Replace Array Subset(array=w360, new element=w361, index=w362) -> (w359:T9[])
          }
        }
        n180 = property class="Tosca"(reference=w326, "Accessors:Adapt.Tracks"=w327) -> (reference out=w325:refnum<class "Parameters.lvclass">)  [unwired: 1 in, 1 out]
      }
      event "Tracks": Value Change {
        n181 = event-data() -> ("NewVal"=w370:i32)  [unwired: 1 in]
        n182 = property class="Tosca"(reference=w367) -> (reference out=w366:refnum<class "Parameters.lvclass">, "Accessors:Adapt.Tracks"=w365:T9[])  [unwired: 1 in, 1 out]
        n183 = Array Size(array=w365) -> (size(s)=w369:i32)
        n184 = Less?(x=w370, y=w369) -> (x < y?=w368:bool)
        n185 = case shown="True" w368 {
          tunnel: [_ string[] ["show track"]] -> w371
          frame False {
          }
          frame True {
          }
        }
      }
      event "Switch after": Value Change {
        n186 = event-data() -> ()  [unwired: 1 in, 1 out]
        n187 = property class="Tosca"(reference=w379) -> (reference out=w376:refnum<class "Parameters.lvclass">, "Accessors:Adapt"=w378:T19)  [unwired: 1 in, 1 out]
        n188 = Bundle By Name(cluster=w378, "Switch after"="Switch after") -> (w375:T19)
        n189 = property class="Tosca"(reference=w376, "Accessors:Adapt"=w375) -> (reference out=w377:refnum<class "Parameters.lvclass">)  [unwired: 1 in, 1 out]
      }
      event "switch type": Value Change {
        n190 = event-data() -> ()  [unwired: 1 in, 1 out]
        n191 = property class="Tosca"(reference=w384) -> (reference out=w387:refnum<class "Parameters.lvclass">, "Accessors:Adapt"=w388:T19)  [unwired: 1 in, 1 out]
        n192 = Bundle By Name(cluster=w388, "Switch type"="switch type") -> (w386:T19)
        n193 = property class="Tosca"(reference=w387, "Accessors:Adapt"=w386) -> (reference out=w383:refnum<class "Parameters.lvclass">)  [unwired: 1 in, 1 out]
      }
      event "Adapt": Value Change {
        n194 = event-data() -> ()  [unwired: 1 in, 1 out]
        n195 = property class="Tosca"(reference=w395) -> (reference out=w393:refnum<class "Parameters.lvclass">, "Accessors:Adapt.Tracks"=w391:T9[])  [unwired: 1 in, 1 out]
        n196 = local read "Tracks"() -> (w401:i32)
        n197 = Unbundle By Name("Adapt") -> ("mode"=w411:enum16{"Add", "Multiply"}, "Ndown"=w410:i32, "Nup"=w409:i32, "Nrev"=w408:i32, "Min"=w407:dbl, "Max"=w406:dbl, "Step"=w405:string, "Start"=w404:dbl, "compute"=w400:enum16{"mean", "median"}, "Ncompute"=w399:i32, "Step2"=w397:string, "change after"=w396:i32)
        n198 = Index Array(array=w391, index=w401) -> (element=w403:T9)
        n199 = To Word Integer(number=w400) -> (16bit integer=w398:i16)
        n200 = Bundle By Name(cluster=w403, "Mode"=w411, "Ndown"=w410, "Nup"=w409, "Nreverse"=w408, "Min"=w407, "Max"=w406, "Step"=w405, "Start"=w404, "compute"=w398, "of last"=w399, "Step2"=w397, "after"=w396) -> (w402:T9)
        n201 = Replace Array Subset(array=w391, new element=w402, index=w401) -> (w392:T9[])
        n202 = property class="Tosca"(reference=w393, "Accessors:Adapt.Tracks"=w392) -> (reference out=w394:refnum<class "Parameters.lvclass">)  [unwired: 1 in, 1 out]
      }
      event "Pcatch": Value Change {
        n203 = event-data() -> ()  [unwired: 1 in, 1 out]
        n204 = property class="Tosca"(reference=w419) -> (reference out=w417:refnum<class "Parameters.lvclass">, "Accessors:Adapt.Tracks"=w416:T9[])  [unwired: 1 in, 1 out]
        n205 = local read "Tracks"() -> (w423:i32)
        n206 = Index Array(array=w416, index=w423) -> (element=w422:T9)
        n207 = Bundle By Name(cluster=w422, "Pcatch"="Pcatch") -> (w421:T9)
        n208 = Replace Array Subset(array=w416, new element=w421, index=w423) -> (w415:T9[])
        n209 = property class="Tosca"(reference=w417, "Accessors:Adapt.Tracks"=w415) -> (reference out=w418:refnum<class "Parameters.lvclass">)  [unwired: 1 in, 1 out]
      }
      event User Event {
        w436 = T20 [] ("appended array")
        n210 = event-data() -> ()  [unwired: 1 in, 1 out]
        n211 = property class="Tosca"(reference=w430) -> (reference out=w429:refnum<class "Parameters.lvclass">, "Accessors:Adapt.Tracks"=w427:T9[])  [unwired: 1 in, 1 out]
        n212 = invoke on="Adapt param" class="KTable (strict)" method="Read Table.vi"("Type of Anything"=w436) -> ("Read Table.vi"=w435:variant)  [unwired: 3 in, 3 out]
        n213 = local read "Tracks"() -> (w440:i32)
        n214 = Variant To Data(type=w436, Variant=w435) -> (data=w437:T20)  [unwired: 1 in, 1 out]
        n215 = Index Array(array=w427, index=w440) -> (element=w439:T9)
        n216 = Index Array(array=w437) -> (element=w434:T21)  [unwired: 1 in]
        n217 = Unbundle(w434) -> ("state"=w433:string, "chan"=w432:string, "param"=w431:string)
        n218 = Bundle By Name(cluster=w439, "state"=w433, "chan"=w432, "param"=w431) -> (w438:T9)
        n219 = Replace Array Subset(array=w427, new element=w438, index=w440) -> (w426:T9[])
        n220 = property class="Tosca"(reference=w429, "Accessors:Adapt.Tracks"=w426) -> (reference out=w428:refnum<class "Parameters.lvclass">)  [unwired: 1 in, 1 out]
      }
      event User Event {
        w450 = T22 [] ("Catch")
        n221 = event-data() -> ()  [unwired: 1 in, 1 out]
        n222 = property class="Tosca"(reference=w447) -> (reference out=w445:refnum<class "Parameters.lvclass">, "Accessors:Adapt.Tracks"=w444:T9[])  [unwired: 1 in, 1 out]
        n223 = invoke on="Catch parameters" class="KTable (strict)" method="Read Table.vi"("Type of Anything"=w450) -> ("Read Table.vi"=w449:variant)  [unwired: 3 in, 3 out]
        n224 = local read "Tracks"() -> (w453:i32)
        n225 = Index Array(array=w444, index=w453) -> (element=w452:T9)
        n226 = Variant To Data(type=w450, Variant=w449) -> (data=w448:T22)  [unwired: 1 in, 1 out]
        n227 = Bundle By Name(cluster=w452, "Catch"=w448) -> (w451:T9)
        n228 = Replace Array Subset(array=w444, new element=w451, index=w453) -> (w443:T9[])
        n229 = property class="Tosca"(reference=w445, "Accessors:Adapt.Tracks"=w443) -> (reference out=w446:refnum<class "Parameters.lvclass">)  [unwired: 1 in, 1 out]
      }
      event User Event {
        w463 = T22 [] ("Catch")
        n230 = event-data() -> ()  [unwired: 1 in, 1 out]
        n231 = property class="Tosca"(reference=w460) -> (reference out=w458:refnum<class "Parameters.lvclass">, "Accessors:Adapt.Tracks"=w456:T9[])  [unwired: 1 in, 1 out]
        n232 = invoke on="Test param" class="KTable (strict)" method="Read Table.vi"("Type of Anything"=w463) -> ("Read Table.vi"=w462:variant)  [unwired: 3 in, 3 out]
        n233 = local read "Tracks"() -> (w466:i32)
        n234 = Index Array(array=w456, index=w466) -> (element=w465:T9)
        n235 = Variant To Data(type=w463, Variant=w462) -> (data=w461:T22)  [unwired: 1 in, 1 out]
        n236 = Bundle By Name(cluster=w465, "Vars"=w461) -> (w464:T9)
        n237 = Replace Array Subset(array=w456, new element=w464, index=w466) -> (w457:T9[])
        n238 = property class="Tosca"(reference=w458, "Accessors:Adapt.Tracks"=w457) -> (reference out=w459:refnum<class "Parameters.lvclass">)  [unwired: 1 in, 1 out]
      }
      event Value Change {
        n239 = event-data() -> ()  [unwired: 1 in, 1 out]
        n240 = property class="Tosca"(reference=w473) -> (reference out=w471:refnum<class "Parameters.lvclass">, "Accessors:Adapt.Tracks"=w469:T9[])  [unwired: 1 in, 1 out]
        n241 = local read "Tracks"() -> (w477:i32)
        n242 = Index Array(array=w469, index=w477) -> (element=w476:T9)
        n243 = Bundle By Name(cluster=w476, "do all catch"="all catch") -> (w475:T9)
        n244 = Replace Array Subset(array=w469, new element=w475, index=w477) -> (w470:T9[])
        n245 = property class="Tosca"(reference=w471, "Accessors:Adapt.Tracks"=w470) -> (reference out=w472:refnum<class "Parameters.lvclass">)  [unwired: 1 in, 1 out]
      }
    }
    n246 = while {
      shift-right: [w488] -> w41
      shift-left: w43 -> [w487]
      shift-right: [w486] -> _
      shift-left: w42 -> [w491]
      tunnel: [w484] -> w40
      tunnel: [w483] -> w39
      shift-right: [w481] -> w36
      shift-left: w37 -> [w482]
      tunnel: w34 -> [w480]
      stop <- w485 stop-if-true
      n247 = Delete From Array(array=w491) -> (deleted portion=w489:string, array with subset deleted=w490:string[])  [unwired: 2 in]
      n248 = case shown="\"script\"" w489 {
        tunnel: w490 -> [w494 w500 w506 w511 w526 w538 w561 w574 w585 w608 w645 w658 w690]
        tunnel: [w494 w500 w506 w511 w526 w537 w561 w574 w585 w607 w645 w651 w690] -> w486
        tunnel: [w493 w499 w505 w508 w519 w534 w559 w565 w576 w609 w643 w649 w662] -> w488
        tunnel: w487 -> [w493 w499 w505 w508 w521 w534 w559 w566 w580 w599 w643 w649 w662]
        tunnel: [_ TRUE TRUE _ _ _ _ _ _ _ _ _ _] -> w484
        tunnel: [_ FALSE TRUE _ _ _ _ _ _ _ _ _ _] -> w483
        tunnel: w482 -> [w492 w497 w503 w509 w522 w536 w560 w570 w583 w601 w644 w657 w689]
        tunnel: [w492 w497 w503 w509 w522 w536 w560 w570 w582 w601 w644 w657 w689] -> w481
        tunnel: w480 -> [_ w495 w501 _ _ _ _ _ _ _ _ _ _]
        frame "", Default {
        }
        frame "exit" {
          n249 = Unregister For Events(event registration refnum=w495) -> ()  [unwired: 1 in, 1 out]
        }
        frame "cancel" {
          n250 = Unregister For Events(event registration refnum=w501) -> ()  [unwired: 1 in, 1 out]
        }
        frame "show families" {
          n251 = property class="Tosca"(reference=w508) -> ("Accessors:Schedule.Families"=w507:T12[])  [unwired: 1 in, 2 out]
          n252 = for {
            tunnel: w507 -> [w516] mode=indexing
            tunnel: [w513] -> w510 mode=indexing
            n253 = Unbundle By Name(w516) -> ("Name"=w515:string, "Number"=w514:i32, "one each"=w512:bool)
            n254 = Bundle("Name"=w515, "Number"=w514, "one each"=w512) -> (w513:T23)  [unwired: 1 in]
          }
          n255 = property on="Family" class="KTable (strict)"("Table"=w510) -> ()  [unwired: 2 in, 2 out]
        }
        frame "read families" {
          w524 = cluster{"Name":string, "Number":i32, bool}[] []
          n256 = property class="Tosca"(reference=w521) -> (reference out=w520:refnum<class "Parameters.lvclass">, "Accessors:Schedule.Families"=w518:T12[])  [unwired: 1 in, 1 out]
          n257 = invoke on="Family" class="KTable (strict)" method="Read Table.vi"("Type of Anything"=w524) -> ("Read Table.vi"=w525:variant)  [unwired: 3 in, 3 out]
          n258 = Variant To Data(type=w524, Variant=w525) -> (data=w523:cluster{"Name":string, "Number":i32, bool}[])  [unwired: 1 in, 1 out]
          n259 = for {
            tunnel: w523 -> [w532] mode=indexing
            tunnel: w518 -> [w529] mode=indexing
            tunnel: [w528] -> w517 mode=indexing
            n260 = Unbundle(w532) -> ("Name"=w531:string, "Number"=w530:i32, w527:bool)
            n261 = Bundle By Name(cluster=w529, "Name"=w531, "Number"=w530, "one each"=w527) -> (w528:T12)
          }
          n262 = property class="Tosca"(reference=w520, "Accessors:Schedule.Families"=w517) -> (reference out=w519:refnum<class "Parameters.lvclass">)  [unwired: 1 in, 1 out]
        }
        frame "show params" {
          n263 = property class="Tosca"(reference=w534) -> ("Accessors:Schedule.Families"=w533:T12[])  [unwired: 1 in, 2 out]
          n264 = local read "Family"() -> (w535:u16)
          n265 = Array Size(array=w533) -> (size(s)=w543:i32)
          n266 = Greater Than 0?(x=w543) -> (x > 0?=w544:bool)
          n267 = In Range and Coerce(upper limit=w543, x=w535, lower limit=0) -> (coerced(x)=w542:i32)  [unwired: 1 out]
          n268 = case shown="True" w544 {
            tunnel: w533 -> [_ w554]
            tunnel: w542 -> [_ w553]
            tunnel: [_ w551] -> w541
            tunnel: [_ w550] -> w540
            tunnel: w538 -> [w546 w548]
            tunnel: [w546 w549] -> w537
            frame False {
            }
            frame True {
              n269 = Index Array(array=w554, index=w553) -> (element=w552:T12)
              n270 = Unbundle By Name(w552) -> ("Name"=w551:string, "Vars"=w550:T13[])
              n271 = Build Array (concatenate)(w548, "show grid") -> (w549:string[])
            }
          }
          n272 = control-ref of="Params"() -> (w539:refnum<vi>)
          n273 = call "Tosca-Schedule Params to Table.vi"("Param Table"=w539, "Name"=w541, "Table"=w540) -> ()  [unwired: 13 in]
        }
        frame "set order" {
          n274 = property class="Tosca"(reference=w559) -> ("Accessors:Schedule"=w558:T16)  [unwired: 1 in, 2 out]
          n275 = Unbundle By Name(w558) -> ("order"=w557:T15)
          n276 = Equal?(x=w557, y=Tosca-Sequence_Order."Arbitrary") -> (x = y?=w555:bool)
          n277 = property on="Script" class="Str"("Visible"=w555) -> ()  [unwired: 2 in, 2 out]
          n278 = property on="browse" class="Bool"("Visible"=w555) -> ()  [unwired: 2 in, 2 out]
        }
        frame "read params" {
          n279 = property class="Tosca"(reference=w566) -> (reference out=w564:refnum<class "Parameters.lvclass">, "Accessors:Schedule.Families"=w563:T12[])  [unwired: 1 in, 1 out]
          n280 = local read "Family"() -> (w573:u16)
          n281 = Index Array(array=w563, index=w573) -> (element=w567:T12)
          n282 = control-ref of="Params"() -> (w571:refnum<vi>)
          n283 = Unbundle By Name(w567) -> ("Vars"=w569:T13[])
          n284 = call "Tosca-Table to Schedule Params.vi"("Table In"=w569, "Param Table"=w571) -> ("Table Out"=w568:T13[])  [unwired: 13 in]
          n285 = Bundle By Name(cluster=w567, "Vars"=w568) -> (w572:T12)
          n286 = Replace Array Subset(array=w563, new element=w572, index=w573) -> (w562:T12[])
          n287 = property class="Tosca"(reference=w564, "Accessors:Schedule.Families"=w562) -> (reference out=w565:refnum<class "Parameters.lvclass">)  [unwired: 1 in, 1 out]
        }
        frame "show grid" {
          n288 = property class="Tosca"(reference=w580) -> (reference out=w577:refnum<class "Parameters.lvclass">, "Accessors:Schedule Mode"=w579:T8, "Accessors:Schedule.Families"=w578:T12[])  [unwired: 1 in, 1 out]
          n289 = local read "Family"() -> (w584:u16)
          n290 = case shown="\"CS+/CS-\"" w579 {
            tunnel: w578 -> [w586 w597]
            tunnel: w584 -> [_ w590]
            tunnel: [w586 w589] -> w575
            tunnel: [_ w588] -> w581
            frame "Seq", Default {
              n291 = property on="Grid" class="IntGraph (strict)"("Visible"=FALSE) -> ()  [unwired: 2 in, 2 out]
            }
            frame "CS+/CS-" {
              n292 = Index Array(array=w597, index=w590) -> (element=w598:T12)
              n293 = call "Tosca-Update CS Mask (new).vi"("Family in"=w598) -> ("labels"=w588:string[][], "Family out"=w596:T12, "XVar"=w595:string, "YVar"=w594:string, "Grid"=w593:i32[][])  [unwired: 10 in]
              n294 = Replace Array Subset(array=w597, new element=w596, index=w590) -> (w589:T12[])
              n295 = property on="Grid" class="IntGraph (strict)"("XScale.NameLbl.Text"=w595, "YScale.NameLbl.Text"=w594, "Value"=w593, "Caption.Text"="", "Visible"=TRUE) -> ()  [unwired: 2 in, 2 out]
            }
          }
          n296 = Bundle By Name(cluster=w583, "labels"=w581) -> (w582:T6)
          n297 = property class="Tosca"(reference=w577, "Accessors:Schedule.Families"=w575) -> (reference out=w576:refnum<class "Parameters.lvclass">)  [unwired: 1 in, 1 out]
        }
        frame "update" {
          n298 = property class="Tosca"(reference=w599) -> ("Accessors:Schedule.Families"=w600:T12[])  [unwired: 1 in, 2 out]
          n299 = call "Tosca-Get Conditional Ring Text.vi"("Tosca"=w599) -> ("States"=w606:string[], "StimChans"=w605:cluster{string[]}[], "Params"=w604:cluster{"Parameter Names":string[]}[][])  [unwired: 12 in]
          n300 = for {
            tunnel: [w615] -> w603 mode=indexing if=w610
            tunnel: w606 -> [w614]
            tunnel: w605 -> [w613]
            tunnel: w604 -> [w612]
            tunnel: w600 -> [w611] mode=indexing
            tunnel: [w610] -> _ mode=indexing
            n301 = call "Tosca-Validate Sequence Family.vi"("Family in"=w611, "States"=w614, "StimChans"=w613, "Params"=w612) -> ("errors"=w615:string, "error"=w610:bool)  [unwired: 8 in, 2 out]
          }
          n302 = Empty Array?(array=w603) -> (empty?=w602:bool)
          n303 = case shown="True" w602 {
            tunnel: [_ w625] -> w607
            tunnel: w599 -> [w618 w624]
            tunnel: [w618 w623] -> w609
            tunnel: w608 -> [_ w621]
            tunnel: w600 -> [_ w622]
            tunnel: w603 -> [w617 _]
            frame False {
              n304 = Concatenate Strings(w617) -> (w620:string)
              n305 = call <vilib>:"Error Cluster From Error Code.vi"("error message (\"\")"=w620, "error code (0)"=5129) -> ("error out"=w616:errorcluster)  [unwired: 7 in]
              n306 = call "Error Handler.vi"("error in (no error)"=w616) -> ()  [unwired: 12 in, 3 out]
            }
            frame True {
              n307 = for {
                tunnel: w622 -> [w639] mode=indexing
                tunnel: [w638] -> w627 mode=indexing
                tunnel: [w637] -> w626
                stop <- w637 stop-if-true
                n308 = call "Tosca-Validate Sequence Expressions.vi"("Family in"=w639) -> ("Family out"=w638:T12, "error out"=w637:errorcluster)  [unwired: 13 in]
              }
              n309 = case shown="No Error" w626 {
                selector: w626 -> [_ w635]
                tunnel: w624 -> [w628 w636]
                tunnel: [w629 w636] -> w623
                tunnel: w627 -> [w630 _]
                tunnel: [w633 _] -> w625
                tunnel: w621 -> [w634 _]
                frame No Error {
                  n310 = property class="Tosca"(reference=w628, "Accessors:Schedule.Families"=w630) -> (reference out=w629:refnum<class "Parameters.lvclass">)  [unwired: 1 in, 1 out]
                  n311 = Build Array (concatenate)(w634, "show grid" ("element"), "show families" ("String")) -> (w633:string[])
                }
                frame Error {
                  n312 = call "Error Handler.vi"("error in (no error)"=w635) -> ()  [unwired: 12 in, 3 out]
                }
              }
            }
          }
        }
        frame "script" {
          n313 = property class="Tosca"(reference=w643) -> ("Accessors:Schedule"=w642:T16)  [unwired: 1 in, 2 out]
          n314 = Unbundle By Name(w642) -> ("order"=w641:T15, "Script"=w640:path)
          n315 = case shown="\"Arbitrary\"" w641 {
            tunnel: w640 -> [_ w647]
            frame "Sequential", Default {
            }
            frame "Arbitrary" {
              n316 = call "Tosca-Execute Schedule Order Script.vi"("Path"=w647) -> ("error out"=w646:errorcluster)  [unwired: 13 in, 1 out]
              n317 = call "Error Handler.vi"("error in (no error)"=w646) -> ()  [unwired: 12 in, 3 out]
            }
          }
        }
        frame "show adapt" {
          n318 = property class="Tosca"(reference=w649) -> ("Accessors:Adapt"=w648:T19)  [unwired: 1 in, 2 out]
          n319 = Unbundle By Name(w648) -> ("Switch after"=w656:i32, "Switch type"=w655:enum16{"Trials", "Reversals"})
          n320 = Unbundle By Name(w648) -> ("Tracks"=w654:T9[])
          n321 = for {
            tunnel: w654 -> [w660] mode=indexing
            tunnel: [w659] -> w653 mode=indexing
            n322 = Unbundle By Name(w660) -> ("name"=w659:string)
          }
          n323 = local write "Switch after"(w656) -> ()
          n324 = local write "switch type"(w655) -> ()
          n325 = property on="Tracks" class="KListboxEx (strict)"("Items"=w653, "Value"=0 ("Tracks")) -> ()  [unwired: 2 in, 2 out]
          n326 = Build Array (concatenate)(w658, "show track") -> (w651:string[])
        }
        frame "show track" {
          n327 = property class="Tosca"(reference=w662) -> ("Accessors:Adapt.Tracks"=w661:T9[])  [unwired: 1 in, 2 out]
          n328 = local read "Tracks"() -> (w671:i32)
          n329 = Index Array(array=w661, index=w671) -> (element=w670:T9)
          n330 = Unbundle By Name(w670) -> ("state"=w673:string, "chan"=w688:string, "param"=w687:string, "Mode"=w683:enum16{"Add", "Multiply"}, "Step"=w682:string, "Start"=w681:dbl, "Min"=w680:dbl, "Max"=w679:dbl, "Nup"=w678:i32, "Ndown"=w677:i32, "Nreverse"=w676:i32, "compute"=w667:T11, "of last"=w665:i32, "Step2"=w664:string, "after"=w663:i32, "Pcatch"=w674:dbl, "do all catch"=w669:bool)
          n331 = Unbundle By Name(w670) -> ("Catch"=w675:T10[], "Vars"=w668:T10[])
          n332 = local write "Pcatch"(w674) -> ()
          n333 = local write "all catch"(w669) -> ()
          n334 = property on="Catch parameters" class="KTable (strict)"("Table"=w675) -> ()  [unwired: 2 in, 2 out]
          n335 = property on="Test param" class="KTable (strict)"("Table"=w668) -> ()  [unwired: 2 in, 2 out]
          n336 = To Word Integer(number=w667) -> (16bit integer=w666:i16)
          n337 = Bundle("state"=w673, "chan"=w688, "param"=w687) -> (w686:T21)  [unwired: 1 in]
          n338 = local read "Adapt"() -> (w685:T2)
          n339 = Bundle By Name(cluster=w685, "mode"=w683, "Step"=w682, "Start"=w681, "Min"=w680, "Max"=w679, "Nup"=w678, "Ndown"=w677, "Nrev"=w676, "compute"=w666, "Ncompute"=w665, "Step2"=w664, "change after"=w663) -> (w684:T2)
          n340 = Build Array(w686) -> (w672:T20)
          n341 = local write "Adapt"(w684) -> ()
          n342 = property on="Adapt param" class="KTable (strict)"("Table"=w672) -> ()  [unwired: 2 in, 2 out]
        }
      }
      n343 = Empty Array?(array=w486) -> (empty?=w485:bool)
    }
  }
  "Canceled?" <- w32
  "Tosca out" <- w3
